vi "Bind Control Caption.vi"(4 "Ignore Past Updates? (F)":bool, 8 "error in (no error)":errorcluster, 9 "Datum Name (\"\"=Use Control Label)":string, 10 "Control Refnum":refnum<vi>, 11 "IViewable in":refnum<class "IViewable.lvclass">) -> (0 "error out":errorcluster, 3 "IViewable out":refnum<class "IViewable.lvclass">)   [LabVIEW 2017, in "IViewable.lvlib" / "IViewable.lvclass"]
doc: "Bind the Caption of a control terminal (control or indicator) to a published string."
uses:
  IViewable.lvclass
  C:/Program Files (x86)/National Instruments/LabVIEW 2017/vi.lib/ActorFramework/Actor/Actor.lvclass
  <vilib>/ActorFramework/Actor/Actor.lvclass/Actor.ctl
  <vilib>/ActorFramework/Message Enqueuer/Message Enqueuer.lvclass/Message Enqueuer.ctl
  SubscriptionPolicy/ValueChangeSubscription/ValueChangeSubscription.lvclass/ValueChangeSubscription.ctl
  IMediator/SubscriptionRequest/SubscriptionRequest.lvclass/SubscriptionRequest.ctl
  IObserver/IObserver Messages/Subscribe Msg/Subscribe Msg.lvclass/Subscribe Msg.ctl
  <vilib>/ActorFramework/Message Enqueuer/Init from Existing Queue.vi
  <vilib>/ActorFramework/Message Enqueuer/Enqueue.vi
  SubscriptionPolicy/ValueChangeSubscription/ValueChangeSubscription.lvclass
  C:/Git/mva-framework/Source/Framework/IMediator/ISubscriptionPolicy/ISubscriptionPolicy.lvclass
  Transport/ControlCaptionBinding/ControlCaptionBinding.lvclass
  C:/Git/mva-framework/Source/Framework/IMediator/ITransport/ITransport.lvclass
  IObserver/IObserver Messages/Subscribe Msg/Subscribe Msg.lvclass
  C:/Program Files (x86)/National Instruments/LabVIEW 2017/vi.lib/ActorFramework/Message/Message.lvclass
  <vilib>/ActorFramework/Message Priority Queue/Priority Enqueue.vi
  <vilib>/ActorFramework/Message Enqueuer/Message Enqueuer.lvclass
  IMediator/SubscriptionRequest/SubscriptionRequest.lvclass
  <vilib>/ActorFramework/Actor/Actor.lvclass
  IMediator/ISubscriptionPolicy/ISubscriptionPolicy.lvclass
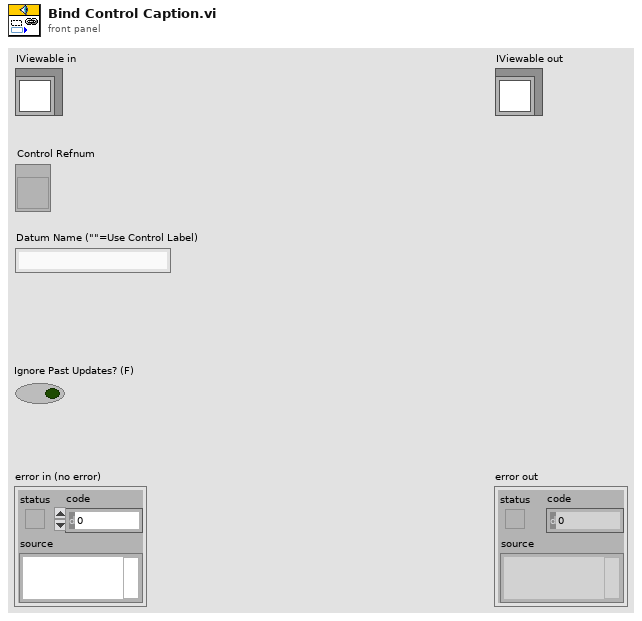
[diagram p1: front panel]
types:
  T1 = typedef "IMediator.lvlib/ISubscriptionPolicy.lvclass/ISubscriptionPolicy Reference.ctl" = refnum<data-value>
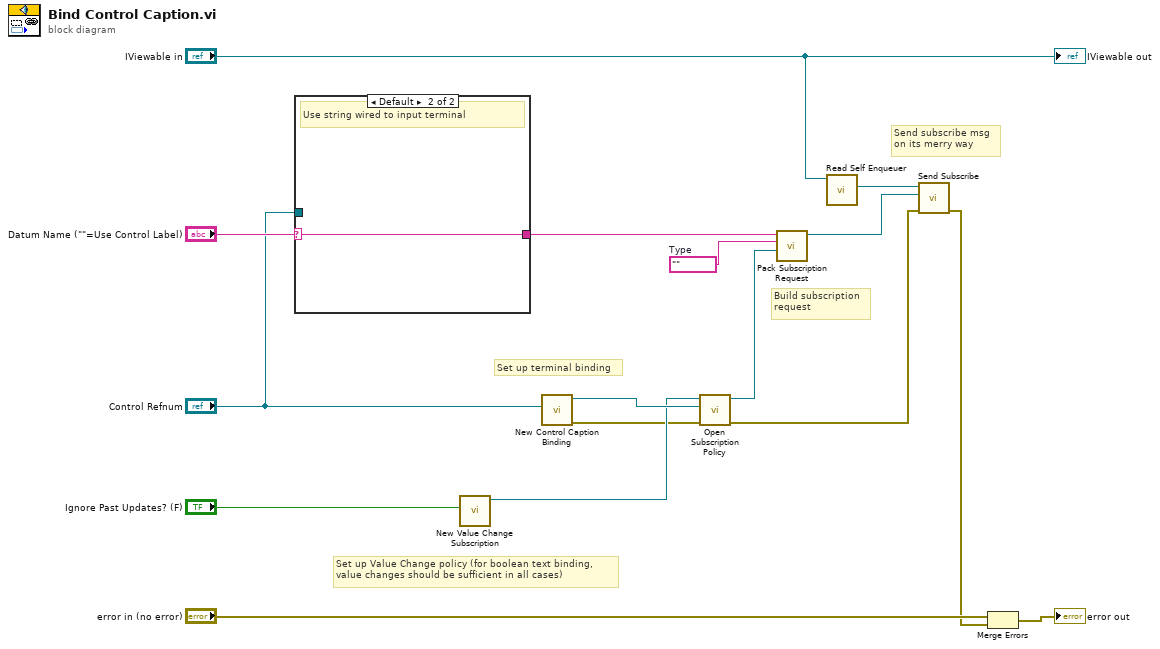
[diagram p0: block diagram]
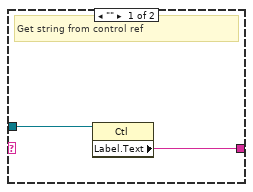
[diagram p2: hidden frame]
diagram:
  w4 = ""  # Type
  # "Set up Value Change policy (for boolean text binding,\nvalue changes should be sufficient in all cases)"
  # "Send subscribe msg\non its merry way"
  # "Build subscription\nrequest"
  # "Set up terminal binding"
  n1 = case shown="Default" "Datum Name (\"\"=Use Control Label)" {
    selector: "Datum Name (\"\"=Use Control Label)" -> [_ w19]
    tunnel: [w17 w19] -> w10
    tunnel: "Control Refnum" -> [w18 _]
    frame "" {
      # "Get string from control ref"
      n2 = property class="Ctl"(reference=w18) -> ("Label.Text"=w17:string)  [unwired: 1 in, 2 out]
    }
    frame Default {
      # "Use string wired to input terminal"
    }
  }
  n3 = call "New Value Change Subscription.vi"("Ignore Past Updates? (F)"="Ignore Past Updates? (F)") -> ("ValueChangeSubscription Out"=w5:refnum<class "ValueChangeSubscription.lvclass">)  [unwired: 10 in]
  n4 = call "New Control Caption Binding.vi"("Ctl Refnum"="Control Refnum") -> ("error out"=w3:errorcluster, "ControlCaptionBinding"=w8:refnum<class "ControlCaptionBinding.lvclass">)  [unwired: 9 in]
  n5 = call "Open Subscription Policy.vi"("error in (no error)"=w3, "Transport"=w8, "SubscriptionPolicy"=w5) -> ("error out"=w2:errorcluster, "Subscription Policy"=w1:T1)  [unwired: 7 in]
  n6 = call "Pack Subscription Request.vi"("Subscription Policy"=w1, "Type"=w4, "Datum Name"=w10) -> ("SubscriptionRequest"=w7:refnum<class "SubscriptionRequest.lvclass">)  [unwired: 8 in]
  n7 = call <vilib>:"Read Self Enqueuer.vi"("Actor"="IViewable in") -> ("Self Enqueuer"=w14:refnum<class "Message Enqueuer.lvclass">)  [unwired: 10 in]
  n8 = call "Send Subscribe.vi"("error in (no error)"=w2, "SubscriptionRequest"=w7, "Message Enqueuer"=w14) -> ("error out"=w12:errorcluster)  [unwired: 7 in, 1 out]
  n9 = Merge Errors("error in (no error)", w12) -> (→"error out":errorcluster)
  "IViewable out" <- "IViewable in"
